vi "SetTempSet.vi"(0 "reference in":refnum<class "Air Conditioner.lvclass">, 2 "TempSet":dbl, 5 "Error In":errorcluster) -> (14 "reference out":refnum<class "Air Conditioner.lvclass">, 19 "Error Out":errorcluster)   [LabVIEW 2024, in "Air Conditioner.lvclass"]
doc: "Accessor methods to TempSet property which presents desired temperature of the room."
uses:
  Air Conditioner.lvclass
  Air Conditioner.lvclass/Air Conditioner.ctl
panel:
  # "Connector Pane"
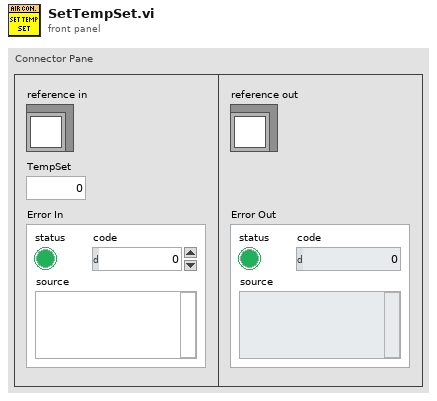
[diagram p1: front panel]
types:
  T1 = typedef "Air Conditioner.lvclass/ObjectAttributes.ctl" = cluster{"State":bool, "TempSet":dbl}
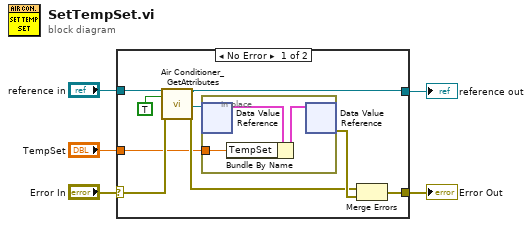
[diagram p0: block diagram]
diagram:
  n1 = case shown="No Error" "Error In" {
    selector: "Error In" -> [w14 w19]
    tunnel: [w11 w19] -> w4
    tunnel: [w9 w18] -> w2
    tunnel: "reference in" -> [w10 w18]
    tunnel: "TempSet" -> [w6 _]
    frame No Error {
      n2 = call "Air Conditioner_GetAttributes.vi"("reference in"=w10, "OnlyGetDvrReference(False)"=TRUE, "Error In"=w14) -> ("reference out"=w9:refnum<class "Air Conditioner.lvclass">, "DataRef"=w7:refnum<data-value>, "Error Out"=w12:errorcluster)  [unwired: 13 in, 1 out]
      n3 = in-place {
        in-place-border: w6 -> [w17]
        n4 = in-place-dvr #1(w7) -> (w16:T1)  [unwired: 1 out]
        n5 = Bundle By Name(cluster=w16, "TempSet"=w17) -> (w15:T1)
        n6 = in-place-dvr #1(w15) -> (w13:errorcluster)  [unwired: 1 out]
      }
      n7 = Merge Errors(w12, w13) -> (w11:errorcluster)
    }
    frame Error {
    }
  }
  "Error Out" <- w4
  "reference out" <- w2
